vi "projectile_motion_1.vi"() -> ()   [LabVIEW 2011]
panel:
  in  "Delta t(sec)":dbl[](array[numeric])=[0.1, 0.05, 0.01]
  out "Waveform Graph":waveform(dbl)[](graph)
  out "XY Graph":cluster{"Y":dbl[], "Y":dbl[]}[](graph)
  in  "Cd*C/m (unitless)":dbl=0.001731
  in  "Stop":bool
  in  "Position_y0":dbl min=0.0
  in  "Position_x0":dbl
  in  "Velocity_0\n(ft/sec)":dbl=147.0
  in  "Angle from Horizon(Degrees)":dbl(knob)=30.0 min=0.0 max=180.0 step=1.0 scale=0.0..180.0
  # "Baseball Graph of Awesomeness"
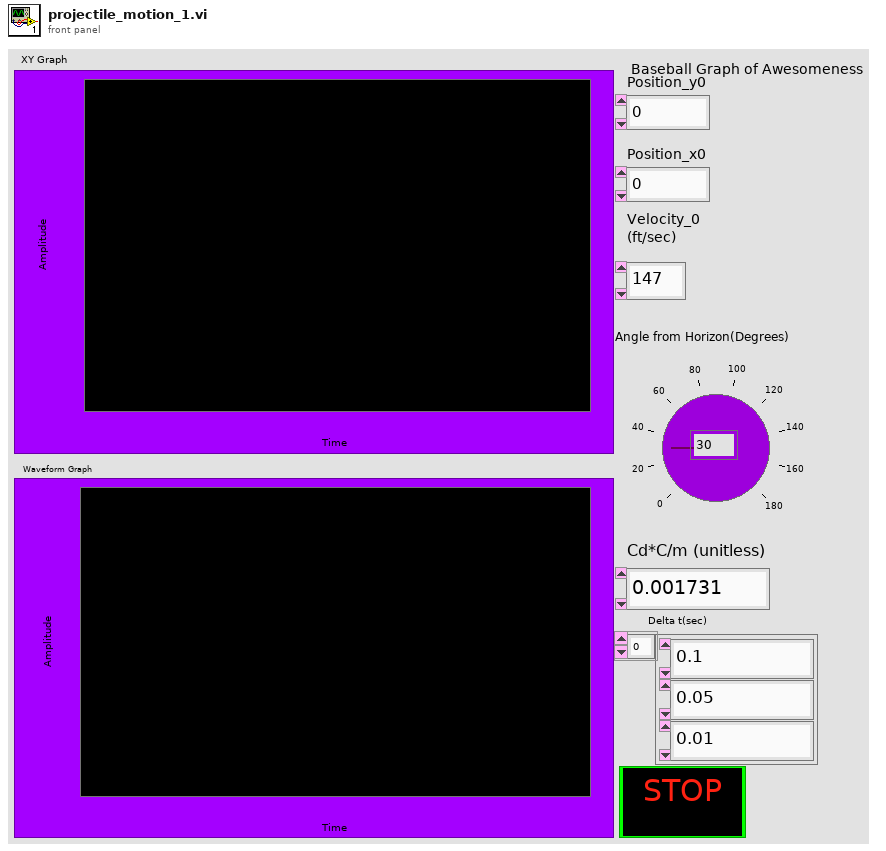
[diagram p1: front panel]
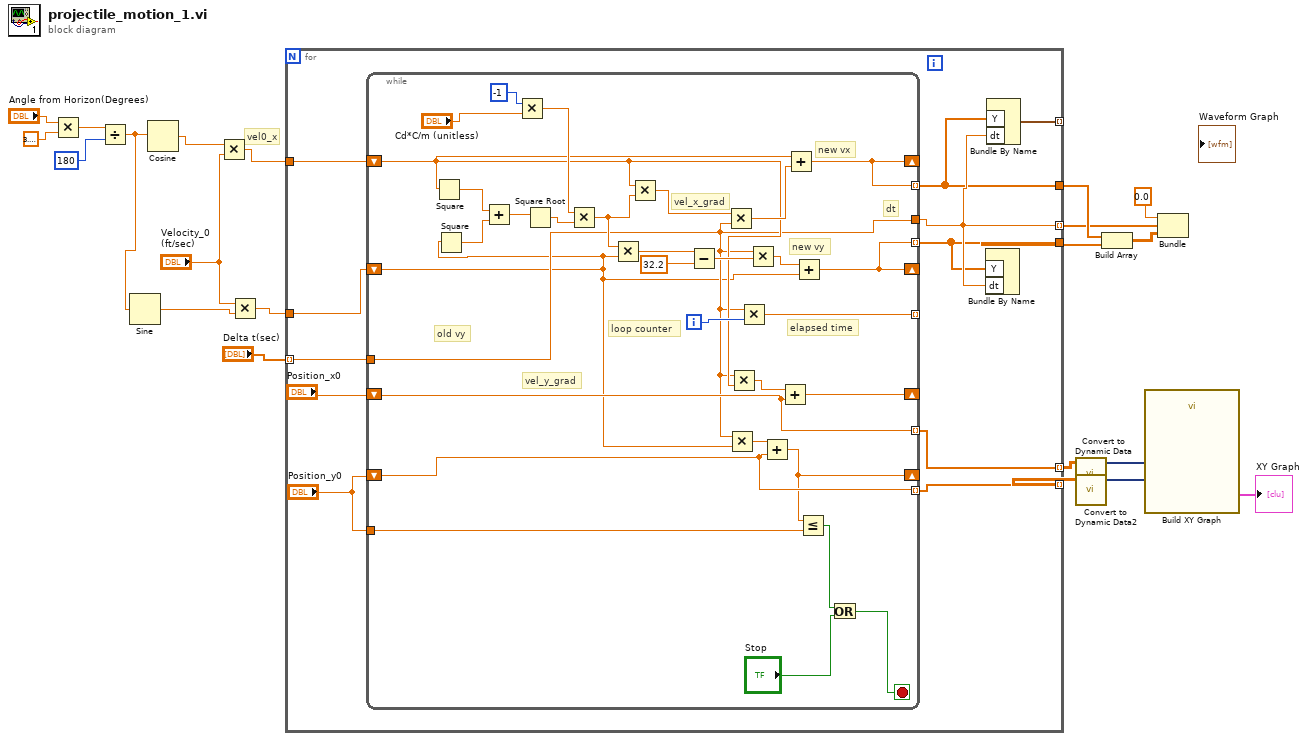
[diagram p0: block diagram]
diagram:
  # "vel0_x"
  n1 = Multiply(x="Angle from Horizon(Degrees)", y=3.141592653589793) -> (x*y=w19:dbl)
  n2 = Divide(x=w19, y=180) -> (x/y=w15:dbl)
  n3 = Sine(x=w15) -> (sin(x)=w13:dbl)
  n4 = Cosine(x=w15) -> (cos(x)=w17:dbl)
  n5 = Multiply(x=w17, y="Velocity_0\n(ft/sec)") -> (x*y=w16:dbl)
  n6 = Multiply(x="Velocity_0\n(ft/sec)", y=w13) -> (x*y=w12:dbl)
  n7 = for {
    tunnel: w16 -> [w32]
    tunnel: w12 -> [w31]
    tunnel: [w28] -> w2 mode=indexing
    tunnel: [w27] -> w10 mode=indexing
    tunnel: [w24] -> w7
    tunnel: [w22] -> w6
    tunnel: "Delta t(sec)" -> [w26] mode=indexing
    tunnel: [w25] -> w4 mode=indexing
    tunnel: [w23] -> _ mode=indexing
    n8 = while {
      tunnel: [w34] -> w25
      tunnel: [w46] -> _ mode=indexing
      tunnel: [w42] -> w28 mode=indexing
      tunnel: "Position_y0" -> [w39]
      tunnel: [w38] -> w27 mode=indexing
      shift-right: [w37] -> _
      shift-left: "Position_y0" -> [w38]
      shift-right: [w43] -> _
      shift-left: "Position_x0" -> [w42]
      shift-right: [w36] -> _
      shift-left: w31 -> [w33]
      tunnel: [w36] -> w22 mode=indexing
      shift-right: [w35] -> _
      shift-left: w32 -> [w45]
      tunnel: [w35] -> w24 mode=indexing
      tunnel: w26 -> [w34]
      i -> [w47]
      stop <- w63 stop-if-true
      # "dt"
      # "new vy"
      # "vel_y_grad"
      # "old vy"
      # "elapsed time"
      # "loop counter"
      # "new vx"
      # "vel_x_grad"
      n9 = Square(x=w45) -> (x^2=w58:dbl)
      n10 = Square(x=w33) -> (x^2=w41:dbl)
      n11 = Add(x=w58, y=w41) -> (x+y=w57:dbl)
      n12 = Multiply(x=-1, y="Cd*C/m (unitless)") -> (x*y=w55:dbl)
      n13 = Square Root(x=w57) -> (sqrt(x)=w56:dbl)
      n14 = Multiply(x=w55, y=w56) -> (x*y=w52:dbl)
      n15 = Multiply(x=w52, y=w33) -> (x*y=w51:dbl)
      n16 = Multiply(x=w45, y=w52) -> (x*y=w53:dbl)
      n17 = Subtract(x=w51, y=32.2) -> (x-y=w49:dbl)
      n18 = Multiply(x=w53, y=w34) -> (x*y=w54:dbl)
      n19 = Multiply(x=w34, y=w33) -> (x*y=w40:dbl)
      n20 = Multiply(x=w34, y=w45) -> (x*y=w44:dbl)
      n21 = Multiply(x=w34, y=w47) -> (x*y=w46:dbl)
      n22 = Multiply(x=w34, y=w49) -> (x*y=w48:dbl)
      n23 = Add(x=w40, y=w38) -> (x+y=w37:dbl)
      n24 = Add(x=w44, y=w42) -> (x+y=w43:dbl)
      n25 = Add(x=w45, y=w54) -> (x+y=w35:dbl)
      n26 = Add(x=w48, y=w33) -> (x+y=w36:dbl)
      n27 = Less Or Equal?(x=w37, y=w39) -> (x <= y?=w61:bool)
      n28 = Or(x=w61, y="Stop") -> (x .or. y?=w63:bool)
    }
    n29 = Bundle By Name("Y"=w22, "dt"=w25) -> ()  [unwired: 1 in, 1 out]
    n30 = Bundle By Name("Y"=w24, "dt"=w25) -> (w23:waveform(dbl))  [unwired: 1 in]
  }
  n31 = call "Convert to Dynamic Data"("2D Array"=w2) -> ("Dynamic Data Type"=w1:dynamicdata)  [unwired: 3 in]
  n32 = call "Convert to Dynamic Data2"("2D Array"=w10) -> ("Dynamic Data Type"=w9:dynamicdata)  [unwired: 3 in]
  n33 = Build Array(w7, w6) -> (w3:dbl[][])
  n34 = call "Build XY Graph"("Y Input"=w9, "X Input"=w1) -> ("XY Graph"=→"XY Graph":cluster{"Y":dbl[], "Y":dbl[]}[])  [unwired: 3 in, 6 out]
  n35 = Bundle(0.0, w4, w3) -> ()  [unwired: 1 in, 1 out]
